vi "Var_serrure.vi"() -> ()   [LabVIEW 2018]
panel:
  in  "MAXE":dbl=5.0
  out "NB_RAND":dbl
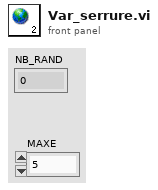
[diagram p1: front panel]
diagram:
